vi "publishJobReport.vi"(8 "error in (no error)":errorcluster, 11 "Job in":refnum<class "Job.lvclass">) -> (0 "error out":errorcluster, 2 "Job Report":T1, 3 "Job out":refnum<class "Job.lvclass">)   [LabVIEW 2013, in "openCron.lvlib" / "Job.lvclass"]
uses:
  Job.lvclass
  Job Report -- cluster.ctl
  Job.lvclass/Job.ctl
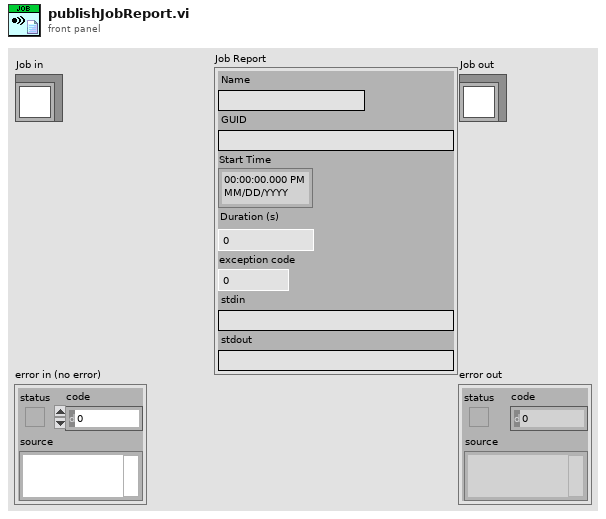
[diagram p1: front panel]
types:
  T1 = typedef "openCron.lvlib/Job.lvclass/Job Report -- cluster.ctl" = cluster{"Name":string, "GUID":string, "Start Time":timestamp, "Duration (s)":dbl, "exception code":i32, "stdin":string, "stdout":string}
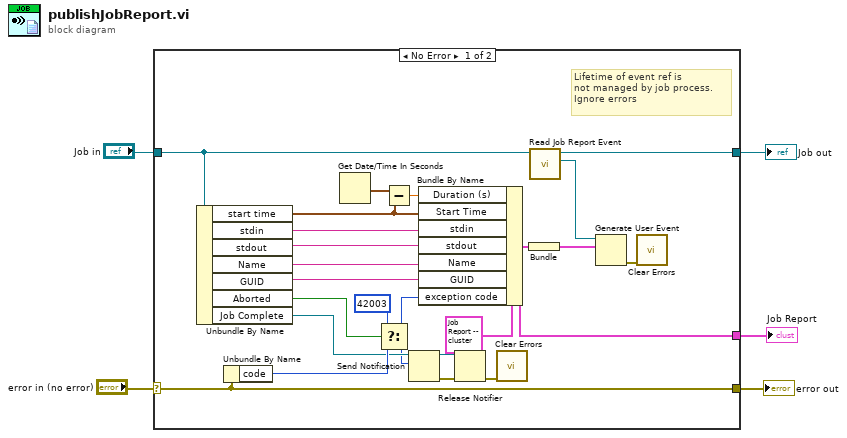
[diagram p0: block diagram]
diagram:
  n1 = case shown="No Error" "error in (no error)" {
    selector: "error in (no error)" -> [w6 w29]
    tunnel: [w21 _] -> w1
    tunnel: "Job in" -> [w15 w30]
    tunnel: [w18 w30] -> w3
    tunnel: [w6 w29] -> w4
    frame No Error {
      # "Lifetime of event ref is\nnot managed by job process. \nIgnore errors"
      n2 = Unbundle By Name(w15) -> ("start time"=w24:timestamp, "stdin"=w14:string, "stdout"=w13:string, "Name"=w28:string, "GUID"=w27:string, "Aborted"=w17:bool, "Job Complete"=w11:refnum<notifier>)
      n3 = Unbundle By Name(w6) -> ("code"=w12:i32)
      n4 = Get Date/Time In Seconds() -> (seconds since 1Jan1904=w25:timestamp)
      n5 = Select(t=42003, s=w17, f=w12) -> (s? t:f=w10:i32)
      n6 = Subtract(x=w25, y=w24) -> (x-y=w23:dbl)
      n7 = Send Notification(notification=w10, notifier=w11) -> (notifier out=w8:refnum<notifier>, error out=w7:errorcluster)  [unwired: 1 in]
      n8 = Bundle By Name(cluster=T1 {"Name"="", "GUID"="", "Start Time"=timestamp(0 s since 1904-01-01), "Duration (s)"=0.0, "exception code"=0, "stdin"="", "stdout"=""} ("Job Report"), "Duration (s)"=w23, "Start Time"=w24, "stdin"=w14, "stdout"=w13, "Name"=w28, "GUID"=w27, "exception code"=w10) -> (w21:T1)
      n9 = Release Notifier(notifier=w8, error in (no error)=w7) -> (error out=w9:errorcluster)  [unwired: 1 in, 2 out]
      n10 = call <vilib>:"Clear Errors.vi"("error in (no error)"=w9) -> ()  [unwired: 6 in, 1 out]
      n11 = Bundle("Job Report"=w21) -> (w20:cluster{"Job Report":T1})  [unwired: 1 in]
      n12 = call "Read Job Report Event.vi"("Job in"=w15) -> ("Job Report Event"=w19:refnum<user-event>, "Job out"=w18:refnum<class "Job.lvclass">)  [unwired: 8 in, 1 out]
      n13 = Generate User Event(user event=w19, event data cluster=w20) -> (error out=w22:errorcluster)  [unwired: 2 in, 1 out]
      n14 = call <vilib>:"Clear Errors.vi"("error in (no error)"=w22) -> ()  [unwired: 6 in, 1 out]
    }
    frame Error {
    }
  }
  "error out" <- w4
  "Job out" <- w3
  "Job Report" <- w1
